vi "scan.vi"() -> ()   [LabVIEW 2017]
uses:
  tools/core/var_config.ctl
  ctrl/var_list.ctl
  tools/analysis/analysis_parameters.ctl
  tools/plotting/plot_element_2D.ctl
  tools/core/generic_config.ctl
  hardware/lecroy/scope_config.ctl
  tools/h5/data_2D.ctl
  tools/analysis/cursors.ctl
  tools/analysis/analysis_result2D.ctl
  tools/core/scan_config.ctl
  <instrlib>/LeCroy Wave Series/Public/Data/Read Multiple Waveforms.vi
  tools/tools.lvlib
  <instrlib>/LeCroy Wave Series/LeCroy Wave Series.lvlib
  hardware/lecroy/lecroy.lvlib
  hardware/highfinesse/highfinesse.lvlib
  <vilib>/gmath/NI_Gmath.lvlib
panel:
  out "state":string
  out "i_chart":dbl(graph)=808.0 caption="index chart"
  in  "preview":bool
  out "v1_chart":dbl(graph) caption="none"
  out "refresh_XY_graph":bool=TRUE
  out "v0_chart":dbl(graph)=644.7000000000019 caption="sirah_shg (nm)"
  out "scope overlay":waveform(dbl)[](graph)
  out "scope data":waveform(dbl)[](graph)
  in  "abort":bool
  in  "pause":bool
  in  "go!":bool
  in  "record":bool=TRUE
  in  "Tab Control":T1(tab)
  in  "exclude":dbl
  in  "plot_lines":bool=TRUE
  in  "sort_by_x":bool caption="sort_x"
  in  "plot_y":T2=enum."f"
  in  "plot_x":T2=enum."v0"
  out "measurement":i32(slide) caption="measurement 508 of 508" scale=0.0..508.0
  out "run_ID":string
  in  "exclude_where_x":bool caption="exclude_x"
  out "v1":dbl caption="none" format="%#_6p"
  out "v0":dbl caption="sirah_shg (nm)" format="%#_6p"
  out "XY Graph":cluster{"sorted_x":dbl[], "sorted_y ":dbl[]}[](graph)
  in  "v0_sort":bool
  in  "test0":bool caption="v0_empty"
  in  "always_update_v0":bool caption="always update?"
  in  "v0_values":dbl[](array[numeric]) format="%#_8p"
  in  "v0_config":T3={"hardware"=enum."none", "options"="", "repeats"=1, "loops"=1, "VISA"="COM9", "override_VISA"=FALSE} {"loops" min=1; "repeats" min=1}
  in  "v0_empty":bool
  in  "v0_build":bool
  in  "v0_shuffle":bool
  in  "v0_load_scan":bool
  in  "v0_save_scan":bool
  in  "v0_func":bool
  in  "v0_inject":bool
  in  "wait_after_v0 (ms)":u32 caption="wait after update (ms)"
  in  "v1_sort":bool
  in  "test1":bool caption="v0_empty"
  in  "always_update_v1":bool caption="always update?"
  in  "v1_config":T3={"hardware"=enum."none", "options"="", "repeats"=1, "loops"=1, "VISA"="COM7", "override_VISA"=FALSE} {"loops" min=1; "repeats" min=1}
  in  "v1_values":dbl[](array[numeric]) format="%#_8p"
  in  "v1_build":bool
  in  "v1_shuffle":bool
  in  "v1_load_scan":bool
  in  "v1_save_scan":bool
  in  "v1_func":bool
  in  "v1_empty":bool
  in  "v1_inject":bool
  in  "wait_after_v1 (ms)":u32 caption="wait after update (ms)"
  in  "source_w1":enum16{"None", "ch1", "ch2", "ch3", "ch4"}(ring)
  in  "source_w0":enum16{"None", "ch1", "ch2", "ch3", "ch4"}(ring)=enum."ch1"
  out "w0_chart":dbl(graph)=644.6808140624936 caption="w0"
  out "w1_chart":dbl(graph)=789.49741 caption="w0"
  in  "export_traces":bool
  in  "get_trace":bool
  out "scope display":waveform(dbl)[](graph)
  out "num_points":i32=2502 caption="points"
  out "dt":dbl=8.000000106811456e-10 format="%#_6p"
  out "num_channels":i32=2 caption="channels"
  out "position":dbl format="%#_6p"
  out "num_overlays":i32=2 caption="overlays"
  in  "wipe overlay":bool
  in  "add overlay":bool
  in  "func":string="a0 - a1" caption="f(a0, a1, a2)"
  out "f_chart":dbl(graph)=-0.0002091954192595339 caption="f (a0, a1, a2)"
  out "a2_chart":dbl(graph)=0.00039806566036490264 caption="a2"
  out "a1_chart":dbl(graph)=-0.0009949684471661708 caption="a1"
  in  "a2":T5={"source"=enum."scope 0", "window"=enum."EF", "type"=enum."mean"}
  in  "a1":T5={"source"=enum."scope 0", "window"=enum."CD", "type"=enum."mean"}
  in  "a0":T5={"source"=enum."scope 0", "window"=enum."AB", "type"=enum."mean"}
  out "a0_chart":dbl(graph)=-0.0012041638664257047 caption="a0"
  in  "scope_config":T6={"scope_VISA"="lecroy", "scope_channels"=[enum."Channel 1"], "timeout (ms)"=100000, "scope_max_points"=2500, "averages"=50} {"averages" min=1; "scope_max_points" items=["50"=50, "100"=100, "250"=250, "500"=500, "1000"=1000, "2500"=2500, "5K"=5000, "10K"=10000, "25K"=25000, "50K"=50000, "100K"=100000, "250K"=250000, "500K"=500000, "1M"=1000000, "2M"=2000000, "2.5M"=2500000, "5M"=5000000, "10M"=10000000, "25M"=25000000, "50M"=50000000, "100M"=100000000]}
  in  "scope_hold_off (ms)":u32=2000 caption="scope hold off (ms)"
  in  "auto_hold":bool=TRUE caption="super_shuffle?"
  in  "var mode":enum16{"permutations", "aligned"}(ring)
  in  "super_shuffle":bool caption="super_shuffle?"
  in  "generic settings":T7={"generic cmd"="", "upper_limit"=5.0, "lower limit"=0.05, "format"="%#.8g"} {"upper_limit" format="%#_13g"}
  in  "trigger rate (Hz)":dbl=25.0
  in  "record_vars":bool=TRUE
  in  "base":path[](array[path])=[path "C:/Users/Adam/scan_data", path "Q:/E11_atmos/scan_data"]
  out "output":path[](array[path])
  out "save_queue":i32
  in  "save_traces":bool=TRUE
  out "queue_full?":bool
  in  "exit":bool
  # "e11 scan"
  # "HighFinesse software must be running"
  # "Configure hardware using \n\n/ctrl/var_master.vi \n\nand the subVIs in \n\n/ctrl/vars"
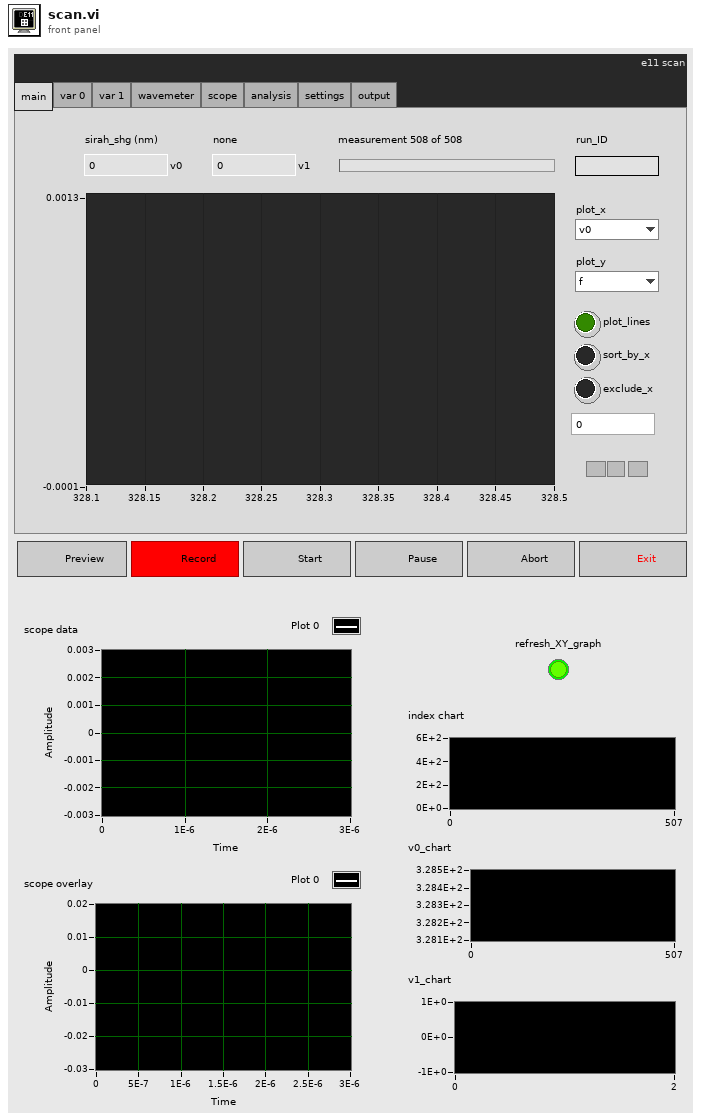
[diagram p1: front panel]
types:
  T1 = enum32{"main", "var 0", "var 1", "wavemeter", "scope", "analysis", "settings", "output"}
  T2 = typedef "tools.lvlib/plot_element_2D.ctl" = enum16{"i", "v0", "v1", "w0", "w1", "a0", "a1", "a2", "f"}
  T3 = typedef "tools.lvlib/var_config.ctl" = cluster{"hardware":T4, "options":string, "repeats":i32, "loops":i32, "VISA":refnum<visa-resource-name>, "override_VISA":bool}
  T4 = typedef "var_list.ctl" = enum16{"none", "AO voltage (V)", "delay (s)", "generic", "microwaves (GHz)", "radiant (nm)", "radiant thg (nm)", "sirah (nm)", "sirah_shg (nm)", "tenma voltage (V)", "wait (s)", "wf_freq (Hz)", "wf_amp (V)", "wf_amp_multi (V)", "wf_offset (V)", "wf_low_level (V)", "wf_high_level (V)", "wf_period (s)", "wf_pulse_width (s)", "wf_sample_rate (Sa/s)", "wf_multi_amp", "wf_multi_freq", "wf_arb_4chan", "WS7 setpoint (nm)"}
  T5 = typedef "tools.lvlib/analysis_parameters.ctl" = cluster{"source":enum16{"scope 0", "scope 1", "scope 2", "scope 3"}, "window":enum16{"AB", "CD", "EF"}, "type":enum16{"sum", "mean", "range"}}
  T6 = typedef "lecroy.lvlib/scope_config.ctl" = cluster{"scope_VISA":refnum<visa-resource-name>, "scope_channels":enum16{"Channel 1", "Channel 2", "Channel 3", "Channel 4"}[], "timeout (ms)":u32, "scope_max_points":i32, "averages":i32}
  T7 = typedef "tools.lvlib/generic_config.ctl" = cluster{"generic cmd":string, "upper_limit":dbl, "lower limit":dbl, "format":string}
  T8 = typedef "tools.lvlib/data_2D.ctl" = cluster{"files":path[], "record":bool, "save traces":bool, "raw data":waveform(dbl)[], "scope_position":dbl, "cursors":T9, "analysis_result":T10, "analysis_pars":T5[], "func":string}
  T9 = typedef "tools.lvlib/cursors.ctl" = cluster{"A":dbl, "B":dbl, "C":dbl, "D":dbl, "E":dbl, "F":dbl}
  T10 = typedef "tools.lvlib/analysis_result2D.ctl" = cluster{"v0":dbl, "v1":dbl, "w0":dbl, "w1":dbl, "a0":dbl, "a1":dbl, "a2":dbl, "f":dbl}
  T11 = enum8{"Enabled", "Disabled", "Disabled and Grayed Out"}
  T12 = enum16{"All Properties", "Averaging", "Interpolation", "Noise Filter", "Invert"}
  T13 = typedef "tools.lvlib/scan_config.ctl" = cluster{"v0 name":string, "v0 num":i32, "v1 name":string, "v1 num":i32, "scan_values":dbl[][], "num rows":i32, "measurement":i32, "v0_config":T3, "v1_config":T3}
  T14 = enum16{"Channel 1", "Channel 2", "Channel 3", "Channel 4"}[]
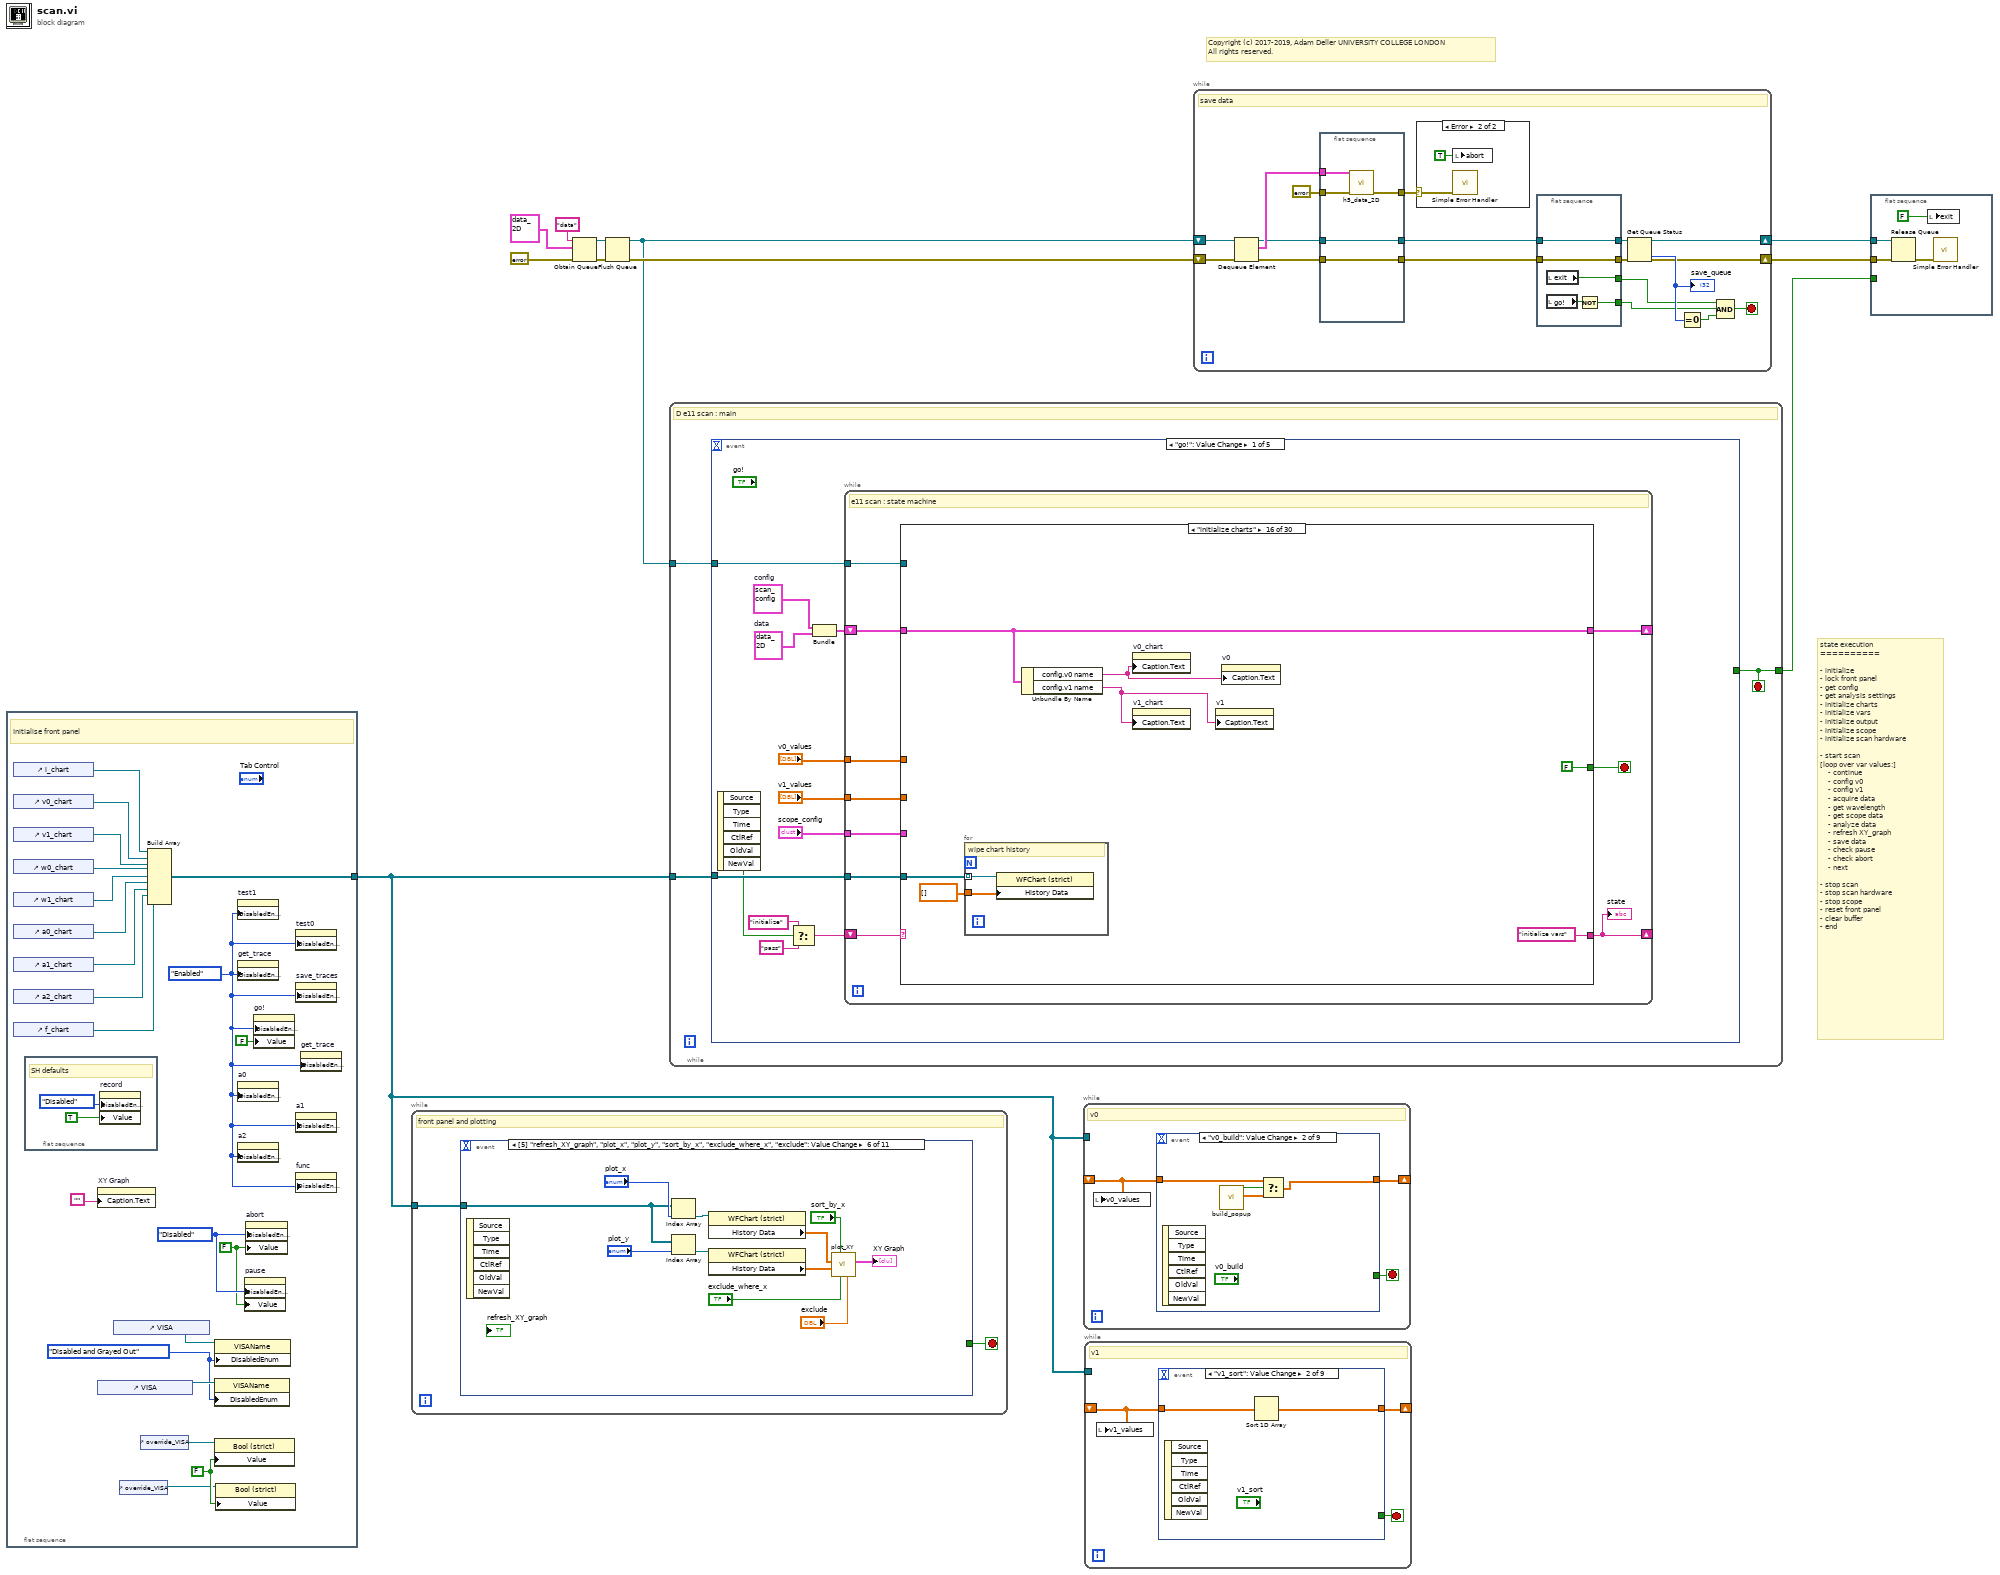
[diagram p0: block diagram]
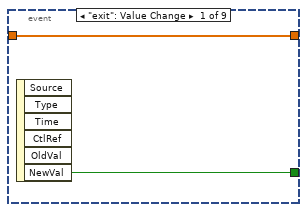
[diagram p2: hidden frame]
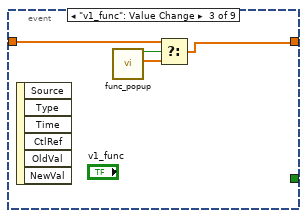
[diagram p3: hidden frame]
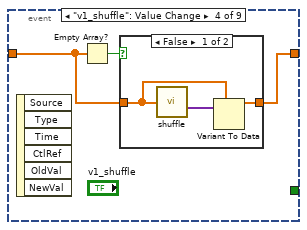
[diagram p4: hidden frame]
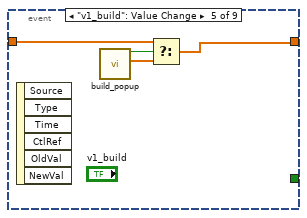
[diagram p6: hidden frame]
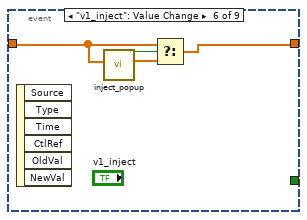
[diagram p7: hidden frame]
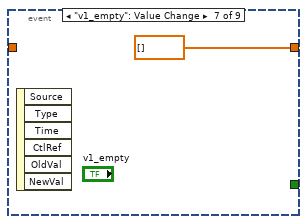
[diagram p8: hidden frame]
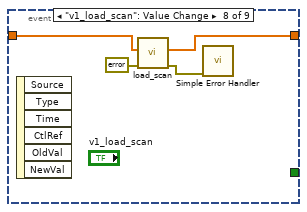
[diagram p9: hidden frame]
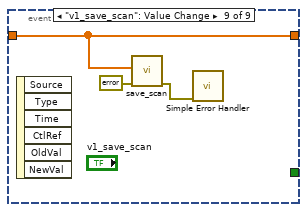
[diagram p10: hidden frame]
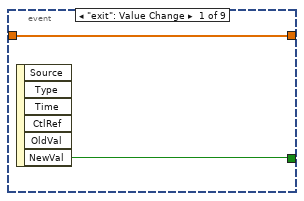
[diagram p11: hidden frame]
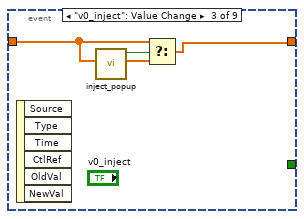
[diagram p12: hidden frame]
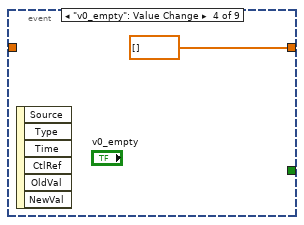
[diagram p13: hidden frame]
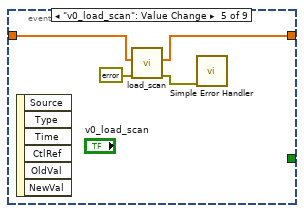
[diagram p14: hidden frame]
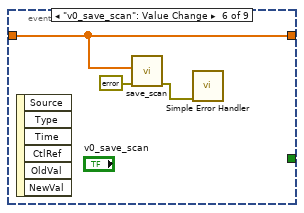
[diagram p15: hidden frame]
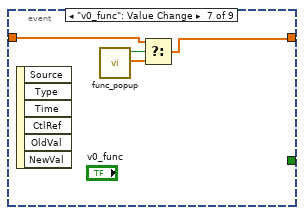
[diagram p16: hidden frame]
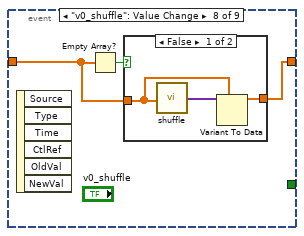
[diagram p17: hidden frame]
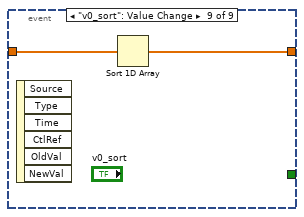
[diagram p19: hidden frame]
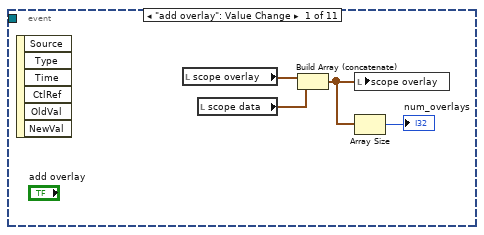
[diagram p20: hidden frame]
diagram:
  # "state execution\n==========\n\n- initialize\n- lock front panel\n- get config\n- get analysis settings\n- initialize charts\n- initialize vars\n- initialize output\n- initialize scope\n- initialize scan hardware\n\n- start scan\n[loop over var values:]\n    - continue\n    - config v0\n    - config v1\n    - acquire data\n    - get wavelength\n    - get scope data\n    - analyze data\n    - refresh XY_graph\n    - save data\n    - check pause\n    - check abort\n    - next\n\n- stop scan\n- stop scan hardware\n- stop scope\n- reset front panel\n- clear buffer\n- end"
  # "Copyright (c) 2017-2019, Adam Deller UNIVERSITY COLLEGE LONDON\nAll rights reserved."
  n1 = flat-sequence {
    tunnel: [w26] -> w1
    frame #0 {
      w17 = FALSE ("Value")
      w14 = T11."Disabled and Grayed Out" ("Disabled")
      w31 = FALSE ("abort")
      w32 = T11."Disabled" ("Disabled")
      w13 = T11."Enabled" ("Disabled")
      # "Initialise front panel"
      n2 = control-ref of="i_chart"() -> (w20:refnum<vi>)
      n3 = control-ref of="v0_chart"() -> (w22:refnum<vi>)
      n4 = control-ref of="v1_chart"() -> (w21:refnum<vi>)
      n5 = control-ref of="w0_chart"() -> (w23:refnum<vi>)
      n6 = control-ref of="w1_chart"() -> (w24:refnum<vi>)
      n7 = control-ref of="a0_chart"() -> (w27:refnum<vi>)
      n8 = control-ref of="a1_chart"() -> (w28:refnum<vi>)
      n9 = control-ref of="a2_chart"() -> (w29:refnum<vi>)
      n10 = control-ref of="f_chart"() -> (w25:refnum<vi>)
      n11 = flat-sequence {
        frame #0 {
          # "SH defaults"
          n12 = property on="record" class="Bool (strict)"("DisabledEnum"=T11."Disabled" ("Disabled"), "Value"=TRUE ("record")) -> ()  [unwired: 2 in, 2 out]
        }
      }
      n13 = property on="XY Graph" class="XYGraph (strict)"("Caption.Text"="") -> ()  [unwired: 2 in, 2 out]
      n14 = control-ref of="VISA"() -> (w15:refnum<vi>)
      n15 = control-ref of="VISA"() -> (w19:refnum<vi>)
      n16 = control-ref of="override_VISA"() -> (w16:refnum<vi>)
      n17 = control-ref of="override_VISA"() -> (w18:refnum<vi>)
      n18 = Build Array(w20, w22, w21, w23, w24, w27, w28, w29, w25) -> (w26:refnum<vi>[])
      n19 = property on="Property Node" class="VISAName"(reference=w15, "DisabledEnum"=w14) -> ()  [unwired: 1 in, 2 out]
      n20 = property on="Property Node" class="Bool (strict)"(reference=w18, "Value"=w17) -> ()  [unwired: 1 in, 2 out]
      n21 = property on="Property Node" class="VISAName"(reference=w19, "DisabledEnum"=w14) -> ()  [unwired: 1 in, 2 out]
      n22 = property on="Property Node" class="Bool (strict)"(reference=w16, "Value"=w17) -> ()  [unwired: 1 in, 2 out]
      n23 = property on="test1" class="Bool"("DisabledEnum"=w13) -> ()  [unwired: 2 in, 2 out]
      n24 = property on="get_trace" class="Bool"("DisabledEnum"=w13) -> ()  [unwired: 2 in, 2 out]
      n25 = property on="a0" class="Clust (strict)"("DisabledEnum"=w13) -> ()  [unwired: 2 in, 2 out]
      n26 = property on="a2" class="Clust (strict)"("DisabledEnum"=w13) -> ()  [unwired: 2 in, 2 out]
      n27 = property on="pause" class="Bool (strict)"("DisabledEnum"=w32, "Value"=w31) -> ()  [unwired: 2 in, 2 out]
      n28 = property on="abort" class="Bool (strict)"("DisabledEnum"=w32, "Value"=w31) -> ()  [unwired: 2 in, 2 out]
      n29 = property on="go!" class="Bool (strict)"("DisabledEnum"=w13, "Value"=FALSE ("go")) -> ()  [unwired: 2 in, 2 out]
      n30 = property on="test0" class="Bool"("DisabledEnum"=w13) -> ()  [unwired: 2 in, 2 out]
      n31 = property on="save_traces" class="Bool (strict)"("DisabledEnum"=w13) -> ()  [unwired: 2 in, 2 out]
      n32 = property on="a1" class="Clust (strict)"("DisabledEnum"=w13) -> ()  [unwired: 2 in, 2 out]
      n33 = property on="func" class="Str"("DisabledEnum"=w13) -> ()  [unwired: 2 in, 2 out]
      n34 = property on="get_trace" class="Bool"("DisabledEnum"=w13) -> ()  [unwired: 2 in, 2 out]
    }
  }
  n35 = while {
    tunnel: w1 -> [w35]
    stop <- w36 stop-if-true
    # "front panel and plotting"
    n36 = event shown="[5] \"refresh_XY_graph\", \"plot_x\", \"plot_y\", \"sort_by_x\", \"exclude_where_x\", \"exclude\": Value Change" {
      selector: _ -> [_ _ _ _ _ _ _ _ _ _ _]
      dyn-events: _ -> [_ _ _ _ _ _ _ _ _ _ _]
      timeout: _ -> [_ _ _ _ _ _ _ _ _ _ _]
      tunnel: [_ w41 _ _ _ _ _ _ _ _ _] -> w36
      tunnel: w35 -> [_ _ _ _ _ w70 _ _ _ _ _]
      event "add overlay": Value Change {
        n37 = event-data() -> ()  [unwired: 1 in, 6 out]
        n38 = local read "scope overlay"() -> (w38:waveform(dbl)[])
        n39 = local read "scope data"() -> (w37:waveform(dbl)[])
        n40 = Build Array (concatenate)(w38, w37) -> (w39:waveform(dbl)[])
        n41 = local write "scope overlay"(w39) -> ()
        n42 = Array Size(array=w39) -> (size(s)=→"num_overlays":i32)
      }
      event "exit": Value Change {
        n43 = event-data() -> ("NewVal"=w41:bool)  [unwired: 1 in, 5 out]
      }
      event "export_traces": Value Change {
        n44 = event-data() -> ()  [unwired: 1 in, 6 out]
        n45 = local read "position"() -> (w44:dbl)
        n46 = local read "scope data"() -> (w45:waveform(dbl)[])
        n47 = call "save_traces.vi"("error in"=errorcluster {"status"=FALSE, "code"=0, "source"=""}, "position"=w44, "data"=w45) -> ("error out"=w43:errorcluster)  [unwired: 8 in]
        n48 = call <vilib>:"Simple Error Handler.vi"("error in (no error)"=w43) -> ()  [unwired: 4 in, 5 out]
      }
      event "plot_lines": Value Change {
        n49 = event-data() -> ()  [unwired: 1 in, 6 out]
        n50 = case shown="True" "plot_lines" {
          tunnel: [u8 0 ("Plot.Line Style") u8 0 ("Plot.Line Style")] -> w47
          tunnel: [u8 0 u8 1 ("Plot.Line Width")] -> w48
          tunnel: [u32 16448250 ("Plot.Fill/Point Color") u32 8289918 ("Plot.Fill/Point Color")] -> w49
          tunnel: [u8 1 ("Plot.Point Style") u8 12 ("Plot.Point Style")] -> w50
          tunnel: [u32 14671839 ("Plot.Plot Color") u32 14671839 ("Plot.Plot Color")] -> w51
          tunnel: [u8 0 ("Plot.Plot Interpolation") u8 2 ("Plot.Plot Interpolation")] -> w52
          frame False {
          }
          frame True {
          }
        }
        n51 = property on="XY Graph" class="XYGraph (strict)"("Plot.Line Style"=w47, "Plot.Line Width"=w48, "Plot.Fill/Pt. Color"=w49, "Plot.Point Style"=w50, "Plot.Plot Color"=w51, "Plot.Plot Interpolation"=w52) -> ()  [unwired: 2 in, 2 out]
      }
      event "preview": Value Change {
        n52 = event-data() -> ()  [unwired: 1 in, 6 out]
        n53 = local read "v0_config"() -> (w65:T3)
        n54 = local read "v0_values"() -> (w66:dbl[])
        n55 = local read "v1_config"() -> (w67:T3)
        n56 = local read "v1_values"() -> (w68:dbl[])
        n57 = local read "var mode"() -> (w69:enum16{"permutations", "aligned"})
        n58 = call "preview_popup.vi"("var mode"=w69, "v1_values"=w68, "v1_config"=w67, "v0_values"=w66, "v0_config"=w65) -> ()  [unwired: 5 in, 2 out]
      }
      event "refresh_XY_graph", "sort_by_x", "exclude_where_x", "exclude": Value Change {
        n59 = event-data() -> ()  [unwired: 1 in, 6 out]
        n60 = Index Array(array=w70, index="plot_x") -> (element=w72:refnum<vi>)
        n61 = Index Array(array=w70, index="plot_y") -> (element=w71:refnum<vi>)
        n62 = property class="WFChart (strict)"(reference=w72) -> ("History Data"=w75:dbl[])  [unwired: 1 in, 2 out]
        n63 = property class="WFChart (strict)"(reference=w71) -> ("History Data"=w76:dbl[])  [unwired: 1 in, 2 out]
        n64 = call "plot_XY.vi"("exclude"="exclude", "exclude_where_x"="exclude_where_x", "sort_by_x"="sort_by_x", "Y_Data"=w76, "X_Data"=w75) -> ("XY Graph"=→"XY Graph":cluster{"sorted_x":dbl[], "sorted_y ":dbl[]}[])  [unwired: 6 in]
      }
      event Value Change {
        n65 = event-data() -> ()  [unwired: 1 in, 6 out]
        n66 = control-ref of="override_VISA"() -> (w82:refnum<vi>)
        n67 = property on="Property Node" class="Bool (strict)"(reference=w82, "Val(Sgnl)"=FALSE ("Value")) -> ()  [unwired: 1 in, 2 out]
      }
      event Value Change {
        n68 = event-data() -> ("NewVal"=w83:bool)  [unwired: 1 in, 5 out]
        n69 = control-ref of="VISA"() -> (w86:refnum<vi>)
        n70 = Select(t=T11."Enabled" ("Disabled"), s=w83, f=T11."Disabled and Grayed Out" ("Disabled")) -> (s? t:f=w87:T11)
        n71 = property on="Property Node" class="VISAName"(reference=w86, "DisabledEnum"=w87) -> ()  [unwired: 1 in, 2 out]
      }
      event Value Change {
        n72 = event-data() -> ()  [unwired: 1 in, 6 out]
        n73 = control-ref of="override_VISA"() -> (w89:refnum<vi>)
        n74 = property on="Property Node" class="Bool (strict)"(reference=w89, "Val(Sgnl)"=FALSE ("Value")) -> ()  [unwired: 1 in, 2 out]
      }
      event Value Change {
        n75 = event-data() -> ("NewVal"=w90:bool)  [unwired: 1 in, 5 out]
        n76 = Select(t=T11."Enabled" ("Disabled"), s=w90, f=T11."Disabled and Grayed Out" ("Disabled")) -> (s? t:f=w94:T11)
        n77 = control-ref of="VISA"() -> (w93:refnum<vi>)
        n78 = property on="Property Node" class="VISAName"(reference=w93, "DisabledEnum"=w94) -> ()  [unwired: 1 in, 2 out]
      }
      event "wipe overlay": Value Change {
        w95 = waveform(dbl)[] [] ("Waveform Data")
        n79 = event-data() -> ()  [unwired: 1 in, 6 out]
        n80 = local read "scope data"() -> (w97:waveform(dbl)[])
        n81 = local write "scope display"(w97) -> ()
        n82 = Array Size(array=w95) -> (size(s)=w96:i32)
        n83 = local write "num_overlays"(w96) -> ()
        "scope overlay" <- w95
      }
    }
  }
  n84 = Obtain Queue(name (unnamed)="data", element data type=T8 {"files"=[], "record"=FALSE, "save traces"=FALSE, "raw data"=[], "scope_position"=0.0, "cursors"={"A"=0.0, "B"=0.0, "C"=0.0, "D"=0.0, "E"=0.0, "F"=0.0}, "analysis_result"={"v0"=0.0, "v1"=0.0, "w0"=0.0, "w1"=0.0, "a0"=0.0, "a1"=0.0, "a2"=0.0, "f"=0.0}, "analysis_pars"=[], "func"="a0 - a1"} ("data"), error in (no error)=errorcluster {"status"=FALSE, "code"=0, "source"=""}) -> (queue out=w8:refnum<queue>, error out=w9:errorcluster)  [unwired: 2 in, 1 out]
  n85 = Flush Queue(queue=w8, error in (no error)=w9) -> (queue out=w5:refnum<queue>, error out=w6:errorcluster)  [unwired: 1 out]
  n86 = while {
    tunnel: w1 -> [w100]
    tunnel: w5 -> [w99]
    tunnel: [w98] -> w2
    stop <- w98 stop-if-true
    # "D e11 scan : main"
    n87 = event shown="[0] \"go!\": Value Change" {
      selector: _ -> [_ _ _ _ _]
      dyn-events: _ -> [_ _ _ _ _]
      timeout: _ -> [_ _ _ _ _]
      tunnel: [_ _ _ _ "exit"] -> w98
      tunnel: w100 -> [w112 _ _ _ _]
      tunnel: w99 -> [w111 _ _ _ w639]
      event "go!": Value Change {
        w105 = T13 {"v0 name"="radiant (nm)", "v0 num"=808, "v1 name"="none", "v1 num"=808, "scan_values"=[], "num rows"=808, "measurement"=0, "v0_config"={"hardware"=enum."radiant (nm)", "options"="", "repeats"=4, "loops"=1, "VISA"="COM9", "override_VISA"=TRUE}, "v1_config"={"hardware"=enum."radiant (nm)", "options"="", "repeats"=4, "loops"=1, "VISA"="COM9", "override_VISA"=TRUE}}  # config
        w107 = T8 {"files"=[], "record"=FALSE, "save traces"=FALSE, "raw data"=[], "scope_position"=0.0, "cursors"={"A"=0.0, "B"=0.0, "C"=0.0, "D"=0.0, "E"=0.0, "F"=0.0}, "analysis_result"={"v0"=0.0, "v1"=0.0, "w0"=0.0, "w1"=0.0, "a0"=0.0, "a1"=0.0, "a2"=0.0, "f"=0.0}, "analysis_pars"=[], "func"="a0 - a1"}  # data
        n88 = event-data() -> ("NewVal"=w110:bool)  [unwired: 1 in, 5 out]
        n89 = Select(t="initialize" ("state"), s=w110, f="pass" ("state")) -> (s? t:f=w101:string)
        n90 = Bundle("config"=w105, "data"=w107) -> (w106:cluster{"config":T13, "data":T8})  [unwired: 1 in]
        n91 = while {
          shift-right: [w115] -> _
          shift-left: w101 -> [w122]
          shift-right: [w120] -> _
          shift-left: w106 -> [w121]
          tunnel: w111 -> [w118]
          tunnel: w112 -> [w117]
          tunnel: "scope_config" -> [w116]
          tunnel: "v0_values" -> [w114]
          tunnel: "v1_values" -> [w113]
          stop <- w119 stop-if-true
          # "e11 scan : state machine"
          n92 = case shown="\"initialize charts\"" w122 {
            tunnel: ["stop scan" ("f") w129 w152 w176 "check abort" ("next") "end" ("f") w213 w248 "config v0" ("f") "" "initialize charts" ("next") "get analysis settings" ("next") w319 w337 "lock front panel" ("f") "initialize vars" ("next") w378 w416 w437 w480 "get config" ("next") w495 "" "save data" ("f") "clear buffer" ("f") "check pause" ("next") "continue" ("f") "stop scan hardware" ("f") "stop scope" ("f") "reset front panel" ("f")] -> w115
            tunnel: w121 -> [w125 w135 w156 w173 w182 w193 w210 w246 w274 w278 w297 w312 w326 w344 w354 w358 w383 w412 w424 w470 w488 w501 w510 w513 w520 w523 w535 w539 w549 w565]
            tunnel: [w125 w135 w155 w173 w182 w193 w218 w254 w274 w278 w296 w303 w325 w341 w353 w358 w373 w412 w423 w473 w488 w500 w510 w513 w520 w523 w534 w539 w549 w565] -> w120
            tunnel: [FALSE ("error?") FALSE ("error?") FALSE ("error?") FALSE ("error?") FALSE ("error?") FALSE ("error?") FALSE ("error?") FALSE ("error?") FALSE ("error?") TRUE ("error?") FALSE ("error?") FALSE ("error?") FALSE ("error?") FALSE ("error?") FALSE ("error?") FALSE ("error?") FALSE ("error?") FALSE ("error?") FALSE ("error?") FALSE ("error?") FALSE ("error?") FALSE ("error?") TRUE ("error?") FALSE ("error?") FALSE ("error?") FALSE ("error?") FALSE ("error?") FALSE ("error?") FALSE ("error?") FALSE ("error?")] -> w119
            tunnel: w118 -> [_ _ _ _ _ _ _ _ _ _ _ _ _ _ _ _ _ _ _ _ _ _ _ _ _ w527 _ _ _ _]
            tunnel: w117 -> [_ _ _ _ _ _ _ _ _ _ _ _ _ _ _ w361 _ _ _ _ _ _ _ _ _ _ _ _ _ _]
            tunnel: w116 -> [_ w128 _ _ _ _ _ _ _ _ _ _ w318 _ _ _ _ _ w429 _ _ _ _ _ _ _ _ _ _ w557]
            tunnel: w114 -> [_ _ _ _ _ _ w199 _ _ _ _ _ _ _ _ _ w370 w409 _ w459 _ _ _ _ _ _ _ _ w543 _]
            tunnel: w113 -> [_ _ _ _ _ _ _ w236 _ _ _ _ _ _ _ _ w369 w407 _ w458 _ _ _ _ _ _ _ _ w542 _]
            frame "abort", Default {
              n93 = local write "abort"(TRUE ("abort")) -> ()
            }
            frame "acquire data" {
              n94 = Unbundle By Name(w128) -> ("scope_VISA"=w127:refnum<visa-resource-name>)
              n95 = local read "scope_hold_off (ms)"() -> (w137:u32)
              n96 = call <instrlib>:"Configure Continuous Acquisition.vi"("error in (no error)"=errorcluster {"status"=FALSE, "code"=0, "source"=""}, "Continuous Acquisition Mode (T: On)"=TRUE, "VISA resource name"=w127) -> ("error out"=w139:errorcluster, "VISA resource name out"=w140:refnum<visa-resource-name>)  [unwired: 7 in]
              n97 = call "clear_sweeps.vi"("error in (no error)"=w139, "VISA resource name"=w140) -> ("error out"=w138:errorcluster)  [unwired: 8 in, 1 out]
              n98 = flat-sequence {
                tunnel: w138 -> [w142]
                tunnel: w137 -> [w143]
                tunnel: [w142] -> w136
                frame #0 {
                  n99 = Wait (ms)(milliseconds to wait=w143) -> ()  [unwired: 1 out]
                }
              }
              n100 = call <vilib>:"Simple Error Handler.vi"("error in (no error)"=w136) -> ("error?"=w130:bool)  [unwired: 4 in, 4 out]
              n101 = Select(t="abort", s=w130, f="get wavelength") -> (s? t:f=w129:string)
            }
            frame "analyze data" {
              n102 = Unbundle By Name(w156) -> ("data.func"=w153:string, "data.raw data"=w157:waveform(dbl)[], "data.analysis_pars"=w159:T5[], "data.cursors"=w149:T9)
              n103 = for {
                tunnel: w159 -> [w172] mode=indexing
                tunnel: [w171] -> w165 mode=indexing
                shift-right: [w169] -> w160
                shift-left: errorcluster {"status"=FALSE, "code"=0, "source"=""} ("error in") -> [w170]
                tunnel: w157 -> [w168]
                tunnel: w149 -> [w167]
                n104 = call "analyse.vi"("cursors"=w167, "error in"=w170, "Raw Data"=w168, "analysis_parameters"=w172) -> ("error out"=w169:errorcluster, "result"=w171:dbl)  [unwired: 6 in]
              }
              n105 = call <vilib>:"Simple Error Handler.vi"("error in (no error)"=w160) -> ("error?"=w145:bool)  [unwired: 4 in, 4 out]
              n106 = Index Array(array=w165) -> (element #1=w163:dbl, element #2=w162:dbl, element #3=w161:dbl)  [unwired: 3 in]
              "a1_chart" <- w162
              "a2_chart" <- w161
              "a0_chart" <- w163
              n107 = call <vilib>:"Eval Multi-Variable Scalar.vi"("error in (no error)"=errorcluster {"status"=FALSE, "code"=0, "source"=""}, "Variables"=string[] ["a0", "a1", "a2"], "X Values"=w165, "formula"=w153) -> ("error out"=w148:errorcluster, "y value"=w158:dbl)
              "f_chart" <- w158
              n108 = call <vilib>:"Simple Error Handler.vi"("error in (no error)"=w148) -> ("error?"=w146:bool)  [unwired: 4 in, 4 out]
              n109 = Bundle By Name(cluster=w156, "data.analysis_result.f"=w158, "data.analysis_result.a0"=w163, "data.analysis_result.a1"=w162, "data.analysis_result.a2"=w161) -> (w155:cluster{"config":T13, "data":T8})
              n110 = Or(x=w146, y=w145) -> (x .or. y?=w144:bool)
              n111 = Select(t="abort" ("next"), s=w144, f="refresh XY_graph" ("next")) -> (s? t:f=w152:string)
            }
            frame "check abort" {
              n112 = local read "exit"() -> (w180:bool)
              n113 = Compound Arithmetic op=OR("abort", w180) -> (w175:bool)
              n114 = Select(t="stop scan", s=w175, f="next" ("next")) -> (s? t:f=w176:string)
            }
            frame "check pause" {
              n115 = case shown="True" "pause" {
                frame False {
                  # "continue"
                }
                frame True {
                  # "wait to unpause or abort"
                  n116 = while {
                    stop <- w185 stop-if-true
                    n117 = local read "pause"() -> (w187:bool)
                    n118 = local read "abort"() -> (w189:bool)
                    n119 = local read "exit"() -> (w190:bool)
                    n120 = Not(x=w187) -> (.not. x?=w186:bool)
                    n121 = Wait (ms)(milliseconds to wait=u32 100) -> ()  [unwired: 1 out]
                    n122 = Compound Arithmetic op=OR(w189, w186, w190) -> (w185:bool)
                  }
                }
              }
            }
            frame "clear buffer" {
              n123 = flat-sequence {
                frame #0 {
                  n124 = Wait (ms)(milliseconds to wait=u32 100) -> ()  [unwired: 1 out]
                }
                frame #1 {
                  n125 = while {
                    stop <- w197 stop-if-true
                    n126 = local read "save_queue"() -> (w196:i32)
                    n127 = Equal To 0?(x=w196) -> (x = 0?=w197:bool)
                    n128 = Wait (ms)(milliseconds to wait=u32 100) -> ()  [unwired: 1 out]
                  }
                }
              }
            }
            frame "config v0" {
              n129 = Empty Array?(array=w199) -> (empty?=w201:bool)
              n130 = Unbundle By Name(w210) -> ("config.scan_values"=w208:dbl[][], "config.measurement"=w206:i32, "config.v0_config"=w204:T3)
              n131 = Not(x=w201) -> (.not. x?=w200:bool)
              n132 = Index Array(array=w208, index (row)=w206, index (col)=0 ("disabled index (col)")) -> (element=w205:dbl)
              n133 = Equal To 0?(x=w206) -> (x = 0?=w222:bool)
              n134 = feedback #1() -> (w211:dbl)  [unwired: 1 in]
              n135 = feedback-in #1(w205) -> ()
              n136 = Not Equal?(x=w205, y=w211) -> (x != y?=w223:bool)
              n137 = Compound Arithmetic op=OR(w223, w222, "always_update_v0") -> (w203:bool)
              n138 = And(x=w203, y=w200) -> (x .and. y?=w202:bool)
              n139 = feedback #2(0.0 ("value OUT")) -> (w219:dbl)
              n140 = case shown="True" w202 {
                tunnel: errorcluster {"status"=FALSE, "code"=0, "source"=""} ("error in (no error)") -> [w225 w231]
                tunnel: [w225 w229] -> w217
                tunnel: [w224 w230] -> w209
                tunnel: w219 -> [w224 _]
                tunnel: w205 -> [_ w227]
                tunnel: w204 -> [_ w226]
                frame False {
                  # "don't update"
                }
                frame True {
                  # "update"
                  n141 = call "var_master.vi"("generic settings"="generic settings", "error IN"=w231, "value IN"=w227, "config"=w226) -> ("error OUT"=w229:errorcluster, "value OUT"=w230:dbl)  [unwired: 6 in]
                  n142 = flat-sequence {
                    tunnel: w229 -> [_]
                    frame #0 {
                      n143 = Wait (ms)(milliseconds to wait="wait_after_v0 (ms)") -> ()  [unwired: 1 out]
                    }
                  }
                }
              }
              "v0" <- w209
              "v0_chart" <- w209
              n144 = feedback-in #2(w209) -> ()
              n145 = call <vilib>:"Simple Error Handler.vi"("error in (no error)"=w217) -> ("error?"=w214:bool)  [unwired: 4 in, 4 out]
              n146 = Bundle By Name(cluster=w210, "data.analysis_result.v0"=w209) -> (w218:cluster{"config":T13, "data":T8})
              n147 = Select(t="abort" ("next"), s=w214, f="config v1") -> (s? t:f=w213:string)
            }
            frame "config v1" {
              n148 = Empty Array?(array=w236) -> (empty?=w235:bool)
              n149 = Unbundle By Name(w246) -> ("config.scan_values"=w245:dbl[][], "config.measurement"=w242:i32, "config.v1_config"=w240:T3)
              n150 = Not(x=w235) -> (.not. x?=w234:bool)
              n151 = Index Array(array=w245, index (row)=w242, index (col)=1 ("disabled index (col)")) -> (element=w239:dbl)
              n152 = Equal To 0?(x=w242) -> (x = 0?=w257:bool)
              n153 = feedback #3() -> (w243:dbl)  [unwired: 1 in]
              n154 = feedback-in #3(w239) -> ()
              n155 = Not Equal?(x=w239, y=w243) -> (x != y?=w258:bool)
              n156 = Compound Arithmetic op=OR(w258, w257, "always_update_v1") -> (w237:bool)
              n157 = And(x=w237, y=w234) -> (x .and. y?=w238:bool)
              n158 = feedback #4(0.0 ("value OUT")) -> (w255:dbl)
              n159 = case shown="True" w238 {
                tunnel: errorcluster {"status"=FALSE, "code"=0, "source"=""} ("error in (no error)") -> [w260 w266]
                tunnel: [w260 w264] -> w253
                tunnel: [w259 w265] -> w251
                tunnel: w255 -> [w259 _]
                tunnel: w240 -> [_ w262]
                tunnel: w239 -> [_ w261]
                frame False {
                  # "don't update"
                }
                frame True {
                  # "update"
                  n160 = local read "generic settings"() -> (w263:T7)
                  n161 = call "var_master.vi"("generic settings"=w263, "error IN"=w266, "value IN"=w261, "config"=w262) -> ("error OUT"=w264:errorcluster, "value OUT"=w265:dbl)  [unwired: 6 in]
                  n162 = flat-sequence {
                    tunnel: w264 -> [_]
                    frame #0 {
                      n163 = Wait (ms)(milliseconds to wait="wait_after_v1 (ms)") -> ()  [unwired: 1 out]
                    }
                  }
                }
              }
              "v1" <- w251
              "v1_chart" <- w251
              n164 = feedback-in #4(w251) -> ()
              n165 = Bundle By Name(cluster=w246, "data.analysis_result.v1"=w251) -> (w254:cluster{"config":T13, "data":T8})
              n166 = call <vilib>:"Simple Error Handler.vi"("error in (no error)"=w253) -> ("error?"=w247:bool)  [unwired: 4 in, 4 out]
              n167 = Select(t="abort" ("next"), s=w247, f="acquire data") -> (s? t:f=w248:string)
            }
            frame "continue" {
              n168 = Unbundle By Name(w274) -> ("config.measurement"=w269:i32, "config.num rows"=w273:i32)
              n169 = To Double Precision Float(number=w269) -> (double precision float=→"i_chart":dbl)
              n170 = Increment(x=w269) -> (x+1=w268:i32)
              "measurement" <- w268
              n171 = Format Into String(format string="measurement %d of %d" ("string (\"\")"), w268, w273) -> (resulting string=w271:string)  [unwired: 2 in, 1 out]
              n172 = property on="measurement" class="Slide (strict)"("Caption.Text"=w271) -> ()  [unwired: 2 in, 2 out]
            }
            frame "end" {
            }
            frame "get analysis settings" {
              n173 = for {
                N: 6 -> [_]
                tunnel: [w299] -> w290 mode=indexing
                i -> [w300]
                # "get cursors"
                n174 = property on="scope display" class="WFGraph (strict)"("Active Cursor"=w300) -> ("Cursor.Cursor X"=w299:dbl)  [unwired: 2 in, 2 out]
              }
              n175 = Index Array(array=w290) -> (element #1=w289:dbl, element #2=w288:dbl, element #3=w287:dbl, element #4=w286:dbl, element #5=w285:dbl, element #6=w284:dbl)  [unwired: 6 in]
              n176 = Bundle(cluster=T9 {"A"=0.0, "B"=0.0, "C"=0.0, "D"=0.0, "E"=0.0, "F"=0.0} ("cursors 2"), "A"=w289, "B"=w288, "C"=w287, "D"=w286, "E"=w285, "F"=w284) -> (w281:T9)
              n177 = Build Array("a0", "a1", "a2") -> (w292:T5[])
              n178 = Bundle By Name(cluster=w297, "data.analysis_pars"=w292, "data.func"="func", "data.cursors"=w281) -> (w296:cluster{"config":T13, "data":T8})
            }
            frame "get config" {
              n179 = Bundle By Name(cluster=w312, "config.v0_config"="v0_config", "config.v1_config"="v1_config") -> (w304:cluster{"config":T13, "data":T8})
              n180 = Unbundle By Name("v0_config") -> ("hardware"=w306:T4)
              n181 = Unbundle By Name("v1_config") -> ("hardware"=w305:T4)
              n182 = property on="hardware" class="Enum (strict)"() -> ("Strings []"=w307:string[])  [unwired: 2 in, 2 out]
              n183 = Index Array(array=w307, index=w306) -> (element=w302:string)
              n184 = Index Array(array=w307, index=w305) -> (element=w301:string)
              n185 = Bundle By Name(cluster=w304, "config.v0 name"=w302, "config.v1 name"=w301) -> (w303:cluster{"config":T13, "data":T8})
            }
            frame "get scope data" {
              n186 = Unbundle By Name(w318) -> ("scope_VISA"=w317:refnum<visa-resource-name>, "scope_channels"=w316:T14, "timeout (ms)"=w315:u32)
              n187 = call-poly <instrlib>:"Read Data.vi"("error in (no error)"=errorcluster {"status"=FALSE, "code"=0, "source"=""}, "Timeout (10000 ms)"=w315, "Channels"=w316, "VISA resource name"=w317) -> ("error out"=w313:errorcluster, "Waveform Data"=w314:waveform(dbl)[])  [unwired: 5 in, 1 out]
              n188 = call <vilib>:"Simple Error Handler.vi"("error in (no error)"=w313) -> ("error?"=w320:bool)  [unwired: 4 in, 4 out]
              n189 = flat-sequence {
                tunnel: w314 -> [_]
                tunnel: [w335] -> w327
                frame #0 {
                  n190 = local read "scope overlay"() -> (w335:waveform(dbl)[])
                }
              }
              n191 = Bundle By Name(cluster=w326, "data.raw data"=w314) -> (w325:cluster{"config":T13, "data":T8})
              n192 = Array Size(array=w314) -> (size(s)=→"num_channels":i32)
              n193 = Index Array(array=w314, index=0) -> (element=w333:waveform(dbl))
              n194 = local write "scope data"(w314) -> ()
              n195 = Unbundle By Name(w333) -> ("Y"=w332:dbl[], "dt"=→"dt":dbl)
              n196 = Array Size(array=w332) -> (size(s)=→"num_points":i32)
              n197 = Build Array (concatenate)(w314, w327) -> (→"scope display":waveform(dbl)[])
              n198 = Select(t="abort" ("next"), s=w320, f="analyze data") -> (s? t:f=w319:string)
            }
            frame "get wavelength" {
              n199 = call "get_wl.vi"("error in (no error)"=errorcluster {"status"=FALSE, "code"=0, "source"=""}, "source"="source_w0") -> ("error out"=w348:errorcluster, "wl"=w343:dbl)  [unwired: 8 in]
              "w0_chart" <- w343
              n200 = call "get_wl.vi"("error in (no error)"=w348, "source"="source_w1") -> ("error out"=w347:errorcluster, "wl"=w342:dbl)  [unwired: 8 in]
              "w1_chart" <- w342
              n201 = Bundle By Name(cluster=w344, "data.analysis_result.w0"=w343, "data.analysis_result.w1"=w342) -> (w341:cluster{"config":T13, "data":T8})
              n202 = call <vilib>:"Simple Error Handler.vi"("error in (no error)"=w347) -> ("error?"=w336:bool)  [unwired: 4 in, 4 out]
              n203 = Select(t="abort" ("next"), s=w336, f="get scope data") -> (s? t:f=w337:string)
            }
            frame "initialize" {
              n204 = Bundle By Name(cluster=w354, "config.scan_values"=dbl[][] [] ("scan_values"), "config.measurement"=0 ("measurement")) -> (w353:cluster{"config":T13, "data":T8})
            }
            frame "initialize charts" {
              n205 = for {
                tunnel: w361 -> [w364] mode=indexing
                tunnel: dbl[] [] ("History Data") -> [w363]
                # "wipe chart history"
                n206 = property class="WFChart (strict)"(reference=w364, "History Data"=w363) -> ()  [unwired: 1 in, 2 out]
              }
              n207 = Unbundle By Name(w358) -> ("config.v0 name"=w356:string, "config.v1 name"=w357:string)
              n208 = property on="v0_chart" class="WFChart (strict)"("Caption.Text"=w356) -> ()  [unwired: 2 in, 2 out]
              n209 = property on="v1_chart" class="WFChart (strict)"("Caption.Text"=w357) -> ()  [unwired: 2 in, 2 out]
              n210 = property on="v1" class="DigNum (strict)"("Caption.Text"=w357) -> ()  [unwired: 2 in, 2 out]
              n211 = property on="v0" class="DigNum (strict)"("Caption.Text"=w356) -> ()  [unwired: 2 in, 2 out]
            }
            frame "initialize output" {
              n212 = Get Date/Time In Seconds() -> (seconds since 1Jan1904=w386:timestamp)
              n213 = call "build_rid_iterating.vi"("ext"="_scan.h5", "error in (no error)"=errorcluster {"status"=FALSE, "code"=0, "source"=""}, "save?"="record", "time stamp"=w386, "base"="base") -> ("error out"=w377:errorcluster, "run ID"=w375:string, "output"=w374:path[])  [unwired: 4 in]
              "run_ID" <- w375
              "output" <- w374
              n214 = call <vilib>:"Simple Error Handler.vi"("error in (no error)"=w377) -> ("error?"=w368:bool)  [unwired: 4 in, 4 out]
              n215 = Bundle By Name(cluster=w383, "data.files"=w374, "data.record"="record", "data.save traces"="save_traces") -> (w373:cluster{"config":T13, "data":T8})
              n216 = Not(x=w368) -> (.not. x?=w366:bool)
              n217 = And(x="record", y=w366) -> (x .and. y?=w365:bool)
              n218 = case shown="True" w365 {
                tunnel: w374 -> [_ w395]
                tunnel: w375 -> [_ w394]
                tunnel: w373 -> [_ w403]
                tunnel: [FALSE ("error?") w402] -> w372
                tunnel: w370 -> [_ w401]
                tunnel: w369 -> [_ w400]
                frame False {
                }
                frame True {
                  n219 = Unbundle By Name(w403) -> ("config.v0 num"=w393:i32, "config.v0_config"=w392:T3, "config.v0 name"=w391:string)
                  n220 = Unbundle By Name(w403) -> ("config.v1 name"=w390:string, "config.v1_config"=w389:T3, "config.v1 num"=w388:i32)
                  n221 = call "h5_init_2D.vi"("files"=w395, "var 0"=w391, "v0_config"=w392, "v0_num"=w393, "RID"=w394, "error in (no error)"=errorcluster {"status"=FALSE, "code"=0, "source"=""}, "var 1"=w390, "v1_config"=w389, "v1_num"=w388) -> ("error out"=w396:errorcluster)  [unwired: 6 in]
                  n222 = call "record_vars.vi"("save?"="record_vars", "error in"=w396, "var1_values"=w400, "var0_values"=w401, "output"=w395) -> ("error out"=w399:errorcluster)  [unwired: 6 in]
                  n223 = call <vilib>:"Simple Error Handler.vi"("error in (no error)"=w399) -> ("error?"=w402:bool)  [unwired: 4 in, 4 out]
                }
              }
              n224 = Or(x=w372, y=w368) -> (x .or. y?=w371:bool)
              n225 = Select(t="abort" ("next"), s=w371, f="initialize scope") -> (s? t:f=w378:string)
            }
            frame "initialize scan hardware" {
              n226 = Unbundle By Name(w412) -> ("config.v0_config"=w410:T3, "config.v1_config"=w408:T3)
              n227 = call "pre_scan.vi"("scan_values"=w409, "error in (no error)"=errorcluster {"status"=FALSE, "code"=0, "source"=""} ("error out"), "config"=w410) -> ("error out"=w404:errorcluster)  [unwired: 8 in]
              n228 = flat-sequence {
                tunnel: w408 -> [w420]
                tunnel: w407 -> [w419]
                tunnel: [w418] -> w406
                tunnel: w404 -> [_]
                frame #0 {
                  n229 = call "pre_scan.vi"("scan_values"=w419, "error in (no error)"=errorcluster {"status"=FALSE, "code"=0, "source"=""} ("error out"), "config"=w420) -> ("error out"=w418:errorcluster)  [unwired: 8 in]
                }
              }
              n230 = Merge Errors(w404, w406) -> (w405:errorcluster)
              n231 = call <vilib>:"Simple Error Handler.vi"("error in (no error)"=w405) -> ("error?"=w413:bool)  [unwired: 4 in, 4 out]
              n232 = Select(t="abort" ("next"), s=w413, f="start scan") -> (s? t:f=w416:string)
            }
            frame "initialize scope" {
              n233 = Unbundle By Name(w429) -> ("scope_max_points"=w425:i32, "scope_channels"=w426:T14, "averages"=w427:i32, "scope_VISA"=w428:refnum<visa-resource-name>)
              n234 = call <instrlib>:"Initialize.vi"("error in (no error)"=errorcluster {"status"=FALSE, "code"=0, "source"=""}, "Reset? (T: Yes)"=FALSE, "VISA resource name"=w428) -> ("error out"=w446:errorcluster, "VISA resource name out"=w445:refnum<visa-resource-name>)  [unwired: 7 in]
              n235 = call "read_position.vi"("error in (no error)"=w446, "VISA resource name"=w445) -> ("error out"=w443:errorcluster, "position (s)"=w422:dbl, "VISA resource name out"=w444:refnum<visa-resource-name>)  [unwired: 7 in]
              "position" <- w422
              n236 = call "auto_hold.vi"("averages"=w427, "trigger rate (Hz)"="trigger rate (Hz)", "hold_off"="scope_hold_off (ms)", "auto_hold"="auto_hold") -> ("hold_off (out)"=w431:u32)  [unwired: 7 in]
              n237 = Bundle By Name(cluster=w424, "data.scope_position"=w422) -> (w423:cluster{"config":T13, "data":T8})
              n238 = for {
                shift-right: [w456] -> w450
                shift-left: w443 -> [w454]
                shift-right: [w455] -> w447
                shift-left: w444 -> [w453]
                tunnel: w427 -> [w451]
                tunnel: w426 -> [w452] mode=indexing
                n239 = call <instrlib>:"Configure Channel Preprocessing.vi"("VISA resource name"=w453, "Channel (0: Channel 1)"=w452, "error in (no error)"=w454, "Sweeps to Average (1)"=w451) -> ("VISA resource name out"=w455:refnum<visa-resource-name>, "error out"=w456:errorcluster)  [unwired: 10 in]
              }
              n240 = local write "scope_hold_off (ms)"(w431) -> ()
              n241 = call "num_points.vi"("error in (no error)"=w450, "Maximum Sample Points (500)"=w425, "VISA resource name"=w447) -> ("error out"=w449:errorcluster, "VISA resource name out"=w448:refnum<visa-resource-name>)  [unwired: 7 in]
              n242 = call <instrlib>:"Configure Continuous Acquisition.vi"("error in (no error)"=w449, "Continuous Acquisition Mode (T: On)"=TRUE, "VISA resource name"=w448) -> ("error out"=w435:errorcluster)  [unwired: 7 in, 1 out]
              n243 = call <vilib>:"Simple Error Handler.vi"("error in (no error)"=w435) -> ("error?"=w434:bool)  [unwired: 4 in, 4 out]
              n244 = Select(t="abort" ("next"), s=w434, f="initialize scan hardware") -> (s? t:f=w437:string)
            }
            frame "initialize vars" {
              n245 = Unbundle By Name(w470) -> ("config.v0_config"=w468:T3, "config.v1_config"=w469:T3)
              n246 = call "scan_array_2D.vi"("v1_config"=w469, "v0_config"=w468, "error in"=errorcluster {"status"=FALSE, "code"=0, "source"=""}, "var mode"="var mode", "v1_values"=w458, "v0_values"=w459) -> ("error in (no error)"=w460:errorcluster, "scan_values"=w478:dbl[][])  [unwired: 4 in]
              n247 = call <vilib>:"Simple Error Handler.vi"("error in (no error)"=w460) -> ("error?"=w464:bool)  [unwired: 4 in, 4 out]
              n248 = Array Size(array=w458) -> (size(s)=w465:i32)
              n249 = Array Size(array=w459) -> (size(s)=w466:i32)
              n250 = case shown="True" "super_shuffle" {
                tunnel: w478 -> [w482 w484]
                tunnel: [w482 w483] -> w463
                frame False {
                }
                frame True {
                  n251 = call "shuffle_2D.vi"("Array IN"=w484) -> ("Array OUT"=w485:variant[][])
                  n252 = Variant To Data(type=w484, Variant=w485) -> (data=w483:dbl[][])  [unwired: 1 in, 1 out]
                }
              }
              n253 = Empty Array?(array=w463) -> (empty?=w462:bool)
              n254 = Array Size(array=w463) -> (size(s)=w474:i32[])
              n255 = Or(x=w462, y=w464) -> (x .or. y?=w461:bool)
              n256 = Index Array(array=w474) -> (element=w472:i32)  [unwired: 1 in]
              n257 = To Double Precision Float(number=w472) -> (double precision float=w471:dbl)
              n258 = Bundle By Name(cluster=w470, "config.scan_values"=w463, "config.num rows"=w472, "config.v0 num"=w466, "config.v1 num"=w465) -> (w473:cluster{"config":T13, "data":T8})
              n259 = property on="measurement" class="Slide (strict)"("Scale.Maximum"=w471, "Scale.Minimum"=0.0 ("Scale.Range:Minimum")) -> ()  [unwired: 2 in, 2 out]
              n260 = Select(t="abort" ("next"), s=w461, f="initialize output") -> (s? t:f=w480:string)
            }
            frame "lock front panel" {
              w489 = T11."Disabled and Grayed Out" ("Disabled")
              w490 = T11."Disabled" ("Disabled")
              w491 = T11."Enabled" ("Disabled")
              n261 = property on="pause" class="Bool (strict)"("DisabledEnum"=w491) -> ()  [unwired: 2 in, 2 out]
              n262 = property on="abort" class="Bool (strict)"("DisabledEnum"=w491) -> ()  [unwired: 2 in, 2 out]
              n263 = property on="go!" class="Bool (strict)"("DisabledEnum"=w490) -> ()  [unwired: 2 in, 2 out]
              n264 = property on="save_traces" class="Bool (strict)"("DisabledEnum"=w490) -> ()  [unwired: 2 in, 2 out]
              n265 = property on="record" class="Bool (strict)"("DisabledEnum"=w490) -> ()  [unwired: 2 in, 2 out]
              n266 = property on="a0" class="Clust (strict)"("DisabledEnum"=w489) -> ()  [unwired: 2 in, 2 out]
              n267 = property on="a2" class="Clust (strict)"("DisabledEnum"=w489) -> ()  [unwired: 2 in, 2 out]
              n268 = property on="test1" class="Bool"("DisabledEnum"=w489) -> ()  [unwired: 2 in, 2 out]
              n269 = property on="get_trace" class="Bool"("DisabledEnum"=w489) -> ()  [unwired: 2 in, 2 out]
              n270 = property on="a1" class="Clust (strict)"("DisabledEnum"=w489) -> ()  [unwired: 2 in, 2 out]
              n271 = property on="func" class="Str"("DisabledEnum"=w489) -> ()  [unwired: 2 in, 2 out]
              n272 = property on="test0" class="Bool"("DisabledEnum"=w489) -> ()  [unwired: 2 in, 2 out]
            }
            frame "next" {
              n273 = Unbundle By Name(w501) -> ("config.measurement"=w496:i32, "config.num rows"=w498:i32)
              n274 = Increment(x=w496) -> (x+1=w499:i32)
              n275 = Less?(x=w499, y=w498) -> (x < y?=w497:bool)
              n276 = case shown="True" w497 {
                tunnel: w501 -> [w503 w508]
                tunnel: [w503 w507] -> w500
                tunnel: w499 -> [_ w506]
                tunnel: [FALSE TRUE] -> w493
                frame False {
                }
                frame True {
                  n277 = Bundle By Name(cluster=w508, "config.measurement"=w506) -> (w507:cluster{"config":T13, "data":T8})
                }
              }
              n278 = Select(t="continue", s=w493, f="stop scan") -> (s? t:f=w495:string)
            }
            frame "pass" {
            }
            frame "refresh XY_graph" {
              n279 = property on="refresh_XY_graph" class="Bool (strict)"("Val(Sgnl)"=TRUE ("Value (Signaling)")) -> ()  [unwired: 2 in, 2 out]
            }
            frame "reset front panel" {
              w516 = FALSE ("go")
              w517 = T11."Disabled" ("Disabled")
              w518 = T11."Enabled" ("Disabled")
              n280 = property on="abort" class="Bool (strict)"("Value"=w516) -> ()  [unwired: 2 in, 2 out]
              n281 = property on="go!" class="Bool (strict)"("Value"=w516) -> ()  [unwired: 2 in, 2 out]
              n282 = property on="pause" class="Bool (strict)"("DisabledEnum"=w517) -> ()  [unwired: 2 in, 2 out]
              n283 = property on="abort" class="Bool (strict)"("DisabledEnum"=w517) -> ()  [unwired: 2 in, 2 out]
              n284 = property on="pause" class="Bool (strict)"("Value"=w516) -> ()  [unwired: 2 in, 2 out]
              n285 = property on="save_traces" class="Bool (strict)"("DisabledEnum"=w518) -> ()  [unwired: 2 in, 2 out]
              n286 = property on="go!" class="Bool (strict)"("DisabledEnum"=w518) -> ()  [unwired: 2 in, 2 out]
              n287 = property on="get_trace" class="Bool"("DisabledEnum"=w518) -> ()  [unwired: 2 in, 2 out]
              n288 = property on="a2" class="Clust (strict)"("DisabledEnum"=w518) -> ()  [unwired: 2 in, 2 out]
              n289 = property on="a0" class="Clust (strict)"("DisabledEnum"=w518) -> ()  [unwired: 2 in, 2 out]
              n290 = property on="test1" class="Bool"("DisabledEnum"=w518) -> ()  [unwired: 2 in, 2 out]
              n291 = property on="test0" class="Bool"("DisabledEnum"=w518) -> ()  [unwired: 2 in, 2 out]
              n292 = property on="a1" class="Clust (strict)"("DisabledEnum"=w518) -> ()  [unwired: 2 in, 2 out]
              n293 = property on="func" class="Str"("DisabledEnum"=w518) -> ()  [unwired: 2 in, 2 out]
            }
            frame "save data" {
              n294 = Unbundle By Name(w523) -> ("data"=w522:T8)
              n295 = Enqueue Element(queue=w527, element=w522, error in (no error)=errorcluster {"status"=FALSE, "code"=0, "source"=""}) -> (error out=w526:errorcluster)  [unwired: 1 in, 2 out]
              n296 = while {
                tunnel: w526 -> [_]
                stop <- w529 continue-if-true
                # "clear buffer"
                n297 = local read "save_queue"() -> (w531:i32)
                n298 = Greater?(x=w531, y=12) -> (0:w529:bool)
                "queue_full?" <- w529
                n299 = case shown="True" w529 {
                  frame False {
                  }
                  frame True {
                    n300 = Wait (ms)(milliseconds to wait=u32 100) -> ()  [unwired: 1 out]
                  }
                }
              }
              n301 = call <vilib>:"Simple Error Handler.vi"("error in (no error)"=w526) -> ()  [unwired: 4 in, 5 out]
            }
            frame "start scan" {
              n302 = Bundle By Name(cluster=w535, "config.measurement"=0 ("measurement")) -> (w534:cluster{"config":T13, "data":T8})
            }
            frame "stop scan" {
            }
            frame "stop scan hardware" {
              n303 = Unbundle By Name(w549) -> ("config.v0_config"=w547:T3, "config.v1_config"=w546:T3)
              n304 = call "post_scan.vi"("values"=w543, "error in (no error)"=errorcluster {"status"=FALSE, "code"=0, "source"=""}, "config"=w547) -> ("error out"=w541:errorcluster)  [unwired: 8 in]
              n305 = flat-sequence {
                tunnel: w546 -> [w555]
                tunnel: [w553] -> w545
                tunnel: w542 -> [w552]
                tunnel: w541 -> [_]
                frame #0 {
                  n306 = call "post_scan.vi"("values"=w552, "error in (no error)"=errorcluster {"status"=FALSE, "code"=0, "source"=""}, "config"=w555) -> ("error out"=w553:errorcluster)  [unwired: 8 in]
                }
              }
              n307 = Merge Errors(w541, w545) -> (w544:errorcluster)
              n308 = call <vilib>:"Simple Error Handler.vi"("error in (no error)"=w544) -> ()  [unwired: 4 in, 5 out]
            }
            frame "stop scope" {
              n309 = Unbundle By Name(w557) -> ("scope_VISA"=w556:refnum<visa-resource-name>)
              n310 = call <instrlib>:"Configure Continuous Acquisition.vi"("error in (no error)"=errorcluster {"status"=FALSE, "code"=0, "source"=""}, "Continuous Acquisition Mode (T: On)"=TRUE, "VISA resource name"=w556) -> ("error out"=w558:errorcluster, "VISA resource name out"=w559:refnum<visa-resource-name>)  [unwired: 7 in]
              n311 = call <instrlib>:"Close.vi"("error in (no error)"=w558, "VISA resource name"=w559) -> ("error out"=w563:errorcluster)  [unwired: 9 in]
              n312 = call <vilib>:"Simple Error Handler.vi"("error in (no error)"=w563) -> ()  [unwired: 4 in, 5 out]
            }
          }
          "state" <- w115
        }
      }
      event "get_trace": Value Change {
        n313 = event-data() -> ()  [unwired: 1 in, 6 out]
        n314 = local read "scope_config"() -> (w599:T6)
        n315 = Unbundle By Name(w599) -> ("scope_channels"=w603:T14, "timeout (ms)"=w602:u32, "scope_max_points"=w601:i32, "scope_VISA"=w600:refnum<visa-resource-name>, "averages"=w570:i32)
        n316 = property on="state" class="Str"(error in=errorcluster {"status"=FALSE, "code"=0, "source"=""} ("error in (no error)"), "Val(Sgnl)"="acquire data" ("Value (Signaling)")) -> (error out=w611:errorcluster)  [unwired: 1 in, 1 out]
        n317 = call <instrlib>:"Initialize.vi"("error in (no error)"=w611, "Reset? (T: Yes)"=FALSE, "VISA resource name"=w600) -> ("error out"=w591:errorcluster, "VISA resource name out"=w592:refnum<visa-resource-name>)  [unwired: 7 in]
        n318 = call "read_position.vi"("error in (no error)"=w591, "VISA resource name"=w592) -> ("error out"=w589:errorcluster, "position (s)"=w593:dbl, "VISA resource name out"=w590:refnum<visa-resource-name>)  [unwired: 7 in]
        n319 = call "num_points.vi"("error in (no error)"=w589, "Maximum Sample Points (500)"=w601, "VISA resource name"=w590) -> ("error out"=w605:errorcluster, "VISA resource name out"=w604:refnum<visa-resource-name>)  [unwired: 7 in]
        n320 = local read "scope_hold_off (ms)"() -> (w568:u32)
        n321 = local write "position"(w593) -> ()
        n322 = local read "trigger rate (Hz)"() -> (w569:dbl)
        n323 = for {
          tunnel: w603 -> [w615] mode=indexing
          shift-right: [w616] -> w606
          shift-left: w604 -> [w619]
          shift-right: [w617] -> w607
          shift-left: w605 -> [w618]
          tunnel: w570 -> [w614]
          n324 = call <instrlib>:"Configure Channel Preprocessing.vi"("VISA resource name"=w619, "Update (0: All Properties)"=T12."Averaging", "Channel (0: Channel 1)"=w615, "error in (no error)"=w618, "Sweeps to Average (1)"=w614) -> ("VISA resource name out"=w616:refnum<visa-resource-name>, "error out"=w617:errorcluster)  [unwired: 9 in]
        }
        n325 = local read "auto_hold"() -> (w567:bool)
        n326 = call "auto_hold.vi"("averages"=w570, "trigger rate (Hz)"=w569, "hold_off"=w568, "auto_hold"=w567) -> ("hold_off (out)"=w566:u32)  [unwired: 7 in]
        n327 = call <instrlib>:"Configure Continuous Acquisition.vi"("error in (no error)"=w607, "Continuous Acquisition Mode (T: On)"=TRUE, "VISA resource name"=w606) -> ("error out"=w585:errorcluster, "VISA resource name out"=w586:refnum<visa-resource-name>)  [unwired: 7 in]
        n328 = call "clear_sweeps.vi"("error in (no error)"=w585, "VISA resource name"=w586) -> ("error out"=w588:errorcluster, "VISA resource name out"=w587:refnum<visa-resource-name>)  [unwired: 8 in]
        n329 = local write "scope_hold_off (ms)"(w566) -> ()
        n330 = flat-sequence {
          tunnel: [w623] -> w582
          tunnel: w588 -> [w623]
          tunnel: w587 -> [w622]
          tunnel: [w622] -> w583
          tunnel: w566 -> [w621]
          frame #0 {
            n331 = Wait (ms)(milliseconds to wait=w621) -> ()  [unwired: 1 out]
          }
        }
        n332 = call-poly <instrlib>:"Read Data.vi"("error in (no error)"=w582, "Timeout (10000 ms)"=w602, "Channels"=w603, "VISA resource name"=w583) -> ("error out"=w608:errorcluster, "Waveform Data"=w609:waveform(dbl)[], "VISA resource name out"=w594:refnum<visa-resource-name>)  [unwired: 5 in]
        n333 = local read "scope overlay"() -> (w597:waveform(dbl)[])
        n334 = flat-sequence {
          tunnel: w609 -> [w613]
          tunnel: [""] -> w610
          frame #0 {
            "scope data" <- w613
          }
        }
        n335 = call <instrlib>:"Configure Continuous Acquisition.vi"("error in (no error)"=w608, "Continuous Acquisition Mode (T: On)"=TRUE, "VISA resource name"=w594) -> ("error out"=w596:errorcluster, "VISA resource name out"=w595:refnum<visa-resource-name>)  [unwired: 7 in]
        n336 = Index Array(array=w609, index=0) -> (element=w578:waveform(dbl))
        n337 = Array Size(array=w609) -> (size(s)=w577:i32)
        n338 = Unbundle By Name(w578) -> ("Y"=w579:dbl[], "dt"=w581:dbl)
        n339 = local write "num_channels"(w577) -> ()
        n340 = call <instrlib>:"Close.vi"("error in (no error)"=w596, "VISA resource name"=w595) -> ("error out"=w584:errorcluster)  [unwired: 9 in]
        n341 = property on="state" class="Str"("Val(Sgnl)"=w610) -> ()  [unwired: 2 in, 2 out]
        n342 = Build Array (concatenate)(w609, w597) -> (w598:waveform(dbl)[])
        n343 = local write "dt"(w581) -> ()
        n344 = Array Size(array=w579) -> (size(s)=w580:i32)
        n345 = call <vilib>:"Simple Error Handler.vi"("error in (no error)"=w584) -> ()  [unwired: 4 in, 5 out]
        n346 = local write "scope display"(w598) -> ()
        n347 = local write "num_points"(w580) -> ()
      }
      event "test0": Value Change {
        n348 = event-data() -> ()  [unwired: 1 in, 6 out]
        n349 = property on="v0_values" class="Arr (strict)"() -> ("Value"=w629:dbl[], "Index Values"=w628:u32[])  [unwired: 2 in, 2 out]
        n350 = local read "generic settings"() -> (w625:T7)
        n351 = local read "v0_config"() -> (w624:T3)
        n352 = Index Array(array=w628) -> (element=w627:u32)  [unwired: 1 in]
        n353 = Index Array(array=w629, index=w627) -> (element=w626:dbl)
        n354 = call "test_popup.vi"("value"=w626, "config"=w624, "generic settings"=w625) -> ()  [unwired: 8 in, 1 out]
      }
      event "test1": Value Change {
        n355 = event-data() -> ()  [unwired: 1 in, 6 out]
        n356 = property on="v1_values" class="Arr (strict)"() -> ("Value"=w635:dbl[], "Index Values"=w634:u32[])  [unwired: 2 in, 2 out]
        n357 = local read "generic settings"() -> (w631:T7)
        n358 = local read "v1_config"() -> (w630:T3)
        n359 = Index Array(array=w634) -> (element=w633:u32)  [unwired: 1 in]
        n360 = Index Array(array=w635, index=w633) -> (element=w632:dbl)
        n361 = call "test_popup.vi"("value"=w632, "config"=w630, "generic settings"=w631) -> ()  [unwired: 8 in, 1 out]
      }
      event "exit": Value Change {
        n362 = event-data() -> ()  [unwired: 1 in, 6 out]
        n363 = Enqueue Element(queue=w639, element=T8 {"files"=[], "record"=FALSE, "save traces"=FALSE, "raw data"=[], "scope_position"=0.0, "cursors"={"A"=0.0, "B"=0.0, "C"=0.0, "D"=0.0, "E"=0.0, "F"=0.0}, "analysis_result"={"v0"=0.0, "v1"=0.0, "w0"=0.0, "w1"=0.0, "a0"=0.0, "a1"=0.0, "a2"=0.0, "f"=0.0}, "analysis_pars"=[], "func"="a0 - a1"}, error in (no error)=errorcluster {"status"=FALSE, "code"=0, "source"=""}) -> (error out=w637:errorcluster)  [unwired: 1 in, 2 out]
        n364 = call <vilib>:"Simple Error Handler.vi"("error in (no error)"=w637) -> ()  [unwired: 4 in, 5 out]
      }
    }
  }
  n365 = while {
    shift-right: [w642] -> _
    shift-left: _ -> [w641]
    tunnel: w1 -> [_]
    stop <- w643 stop-if-true
    # "v0"
    n366 = local write "v0_values"(w641) -> ()
    n367 = event shown="[1] \"v0_build\": Value Change" {
      selector: _ -> [_ _ _ _ _ _ _ _ _]
      dyn-events: _ -> [_ _ _ _ _ _ _ _ _]
      timeout: _ -> [_ _ _ _ _ _ _ _ _]
      tunnel: [w645 _ _ _ _ _ _ _ _] -> w643
      tunnel: [w644 w646 w650 dbl[] [] ("v0_values") w657 w659 w662 w666 w673] -> w642
      tunnel: w641 -> [w644 w647 w651 _ w658 w659 w665 w667 w674]
      event "exit": Value Change {
        n368 = event-data() -> ("NewVal"=w645:bool)  [unwired: 1 in, 5 out]
      }
      event "v0_build": Value Change {
        n369 = event-data() -> ()  [unwired: 1 in, 6 out]
        n370 = call "build_popup.vi"() -> ("y_vals"=w648:dbl[], "cancelled"=w649:bool)  [unwired: 10 in]
        n371 = Select(t=w647, s=w649, f=w648) -> (s? t:f=w646:dbl[])
      }
      event "v0_inject": Value Change {
        n372 = event-data() -> ()  [unwired: 1 in, 6 out]
        n373 = call "inject_popup.vi"("y_vals_IN"=w651) -> ("y_vals"=w653:dbl[], "cancelled"=w652:bool)  [unwired: 9 in]
        n374 = Select(t=w651, s=w652, f=w653) -> (s? t:f=w650:dbl[])
      }
      event "v0_empty": Value Change {
        n375 = event-data() -> ()  [unwired: 1 in, 6 out]
      }
      event "v0_load_scan": Value Change {
        n376 = event-data() -> ()  [unwired: 1 in, 6 out]
        n377 = call "load_scan.vi"("error in"=errorcluster {"status"=FALSE, "code"=0, "source"=""}, "values in"=w658) -> ("error out"=w656:errorcluster, "values out"=w657:dbl[])  [unwired: 8 in]
        n378 = call <vilib>:"Simple Error Handler.vi"("error in (no error)"=w656) -> ()  [unwired: 4 in, 5 out]
      }
      event "v0_save_scan": Value Change {
        n379 = event-data() -> ()  [unwired: 1 in, 6 out]
        n380 = call "save_scan.vi"("error in"=errorcluster {"status"=FALSE, "code"=0, "source"=""}, "values in"=w659) -> ("error out"=w660:errorcluster)  [unwired: 9 in]
        n381 = call <vilib>:"Simple Error Handler.vi"("error in (no error)"=w660) -> ()  [unwired: 4 in, 5 out]
      }
      event "v0_func": Value Change {
        n382 = event-data() -> ()  [unwired: 1 in, 6 out]
        n383 = call "func_popup.vi"() -> ("y_vals"=w663:dbl[], "cancelled"=w664:bool)  [unwired: 10 in]
        n384 = Select(t=w665, s=w664, f=w663) -> (s? t:f=w662:dbl[])
      }
      event "v0_shuffle": Value Change {
        n385 = event-data() -> ()  [unwired: 1 in, 6 out]
        n386 = Empty Array?(array=w667) -> (empty?=w668:bool)
        n387 = case shown="False" w668 {
          tunnel: w667 -> [w670 w672]
          tunnel: [w669 w672] -> w666
          frame False {
            n388 = call "shuffle.vi"("Array IN"=w670) -> ("Array OUT"=w671:variant[])
            n389 = Variant To Data(type=w670, Variant=w671) -> (data=w669:dbl[])  [unwired: 1 in, 1 out]
          }
          frame True {
          }
        }
      }
      event "v0_sort": Value Change {
        n390 = event-data() -> ()  [unwired: 1 in, 6 out]
        n391 = Sort 1D Array(array=w674) -> (sorted array=w673:dbl[])
      }
    }
  }
  n392 = while {
    shift-right: [w675] -> _
    shift-left: _ -> [w676]
    tunnel: w1 -> [_]
    stop <- w677 stop-if-true
    # "v1"
    n393 = local write "v1_values"(w676) -> ()
    n394 = event shown="[1] \"v1_sort\": Value Change" {
      selector: _ -> [_ _ _ _ _ _ _ _ _]
      dyn-events: _ -> [_ _ _ _ _ _ _ _ _]
      timeout: _ -> [_ _ _ _ _ _ _ _ _]
      tunnel: [w679 _ _ _ _ _ _ _ _] -> w677
      tunnel: w676 -> [w678 w681 w685 w687 w694 w698 _ w703 w706]
      tunnel: [w678 w680 w682 w686 w693 w697 dbl[] [] ("v1_values") w702 w706] -> w675
      event "exit": Value Change {
        n395 = event-data() -> ("NewVal"=w679:bool)  [unwired: 1 in, 5 out]
      }
      event "v1_sort": Value Change {
        n396 = event-data() -> ()  [unwired: 1 in, 6 out]
        n397 = Sort 1D Array(array=w681) -> (sorted array=w680:dbl[])
      }
      event "v1_func": Value Change {
        n398 = event-data() -> ()  [unwired: 1 in, 6 out]
        n399 = call "func_popup.vi"() -> ("y_vals"=w684:dbl[], "cancelled"=w683:bool)  [unwired: 10 in]
        n400 = Select(t=w685, s=w683, f=w684) -> (s? t:f=w682:dbl[])
      }
      event "v1_shuffle": Value Change {
        n401 = event-data() -> ()  [unwired: 1 in, 6 out]
        n402 = Empty Array?(array=w687) -> (empty?=w688:bool)
        n403 = case shown="False" w688 {
          tunnel: w687 -> [w690 w692]
          tunnel: [w689 w692] -> w686
          frame False {
            n404 = call "shuffle.vi"("Array IN"=w690) -> ("Array OUT"=w691:variant[])
            n405 = Variant To Data(type=w690, Variant=w691) -> (data=w689:dbl[])  [unwired: 1 in, 1 out]
          }
          frame True {
          }
        }
      }
      event "v1_build": Value Change {
        n406 = event-data() -> ()  [unwired: 1 in, 6 out]
        n407 = call "build_popup.vi"() -> ("y_vals"=w696:dbl[], "cancelled"=w695:bool)  [unwired: 10 in]
        n408 = Select(t=w694, s=w695, f=w696) -> (s? t:f=w693:dbl[])
      }
      event "v1_inject": Value Change {
        n409 = event-data() -> ()  [unwired: 1 in, 6 out]
        n410 = call "inject_popup.vi"("y_vals_IN"=w698) -> ("y_vals"=w700:dbl[], "cancelled"=w699:bool)  [unwired: 9 in]
        n411 = Select(t=w698, s=w699, f=w700) -> (s? t:f=w697:dbl[])
      }
      event "v1_empty": Value Change {
        n412 = event-data() -> ()  [unwired: 1 in, 6 out]
      }
      event "v1_load_scan": Value Change {
        n413 = event-data() -> ()  [unwired: 1 in, 6 out]
        n414 = call "load_scan.vi"("error in"=errorcluster {"status"=FALSE, "code"=0, "source"=""}, "values in"=w703) -> ("error out"=w705:errorcluster, "values out"=w702:dbl[])  [unwired: 8 in]
        n415 = call <vilib>:"Simple Error Handler.vi"("error in (no error)"=w705) -> ()  [unwired: 4 in, 5 out]
      }
      event "v1_save_scan": Value Change {
        n416 = event-data() -> ()  [unwired: 1 in, 6 out]
        n417 = call "save_scan.vi"("error in"=errorcluster {"status"=FALSE, "code"=0, "source"=""}, "values in"=w706) -> ("error out"=w707:errorcluster)  [unwired: 9 in]
        n418 = call <vilib>:"Simple Error Handler.vi"("error in (no error)"=w707) -> ()  [unwired: 4 in, 5 out]
      }
    }
  }
  n419 = while {
    shift-right: [w721] -> w3
    shift-left: w5 -> [w724]
    shift-right: [w720] -> w4
    shift-left: w6 -> [w725]
    stop <- w719 stop-if-true
    # "save data"
    n420 = Dequeue Element(queue=w724, error in (no error)=w725) -> (queue out=w714:refnum<queue>, element=w715:T8, error out=w711:errorcluster)  [unwired: 1 in, 1 out]
    n421 = flat-sequence {
      tunnel: w715 -> [w730]
      tunnel: w714 -> [w733]
      tunnel: [w733] -> w713
      tunnel: [w732] -> w712
      tunnel: w711 -> [w732]
      tunnel: errorcluster {"status"=FALSE, "code"=0, "source"=""} ("error in (no error)") -> [w731]
      tunnel: [w729] -> w709
      frame #0 {
        n422 = call "h5_data_2D.vi"("error in (no error)"=w731, "data"=w730) -> ("error out"=w729:errorcluster)  [unwired: 9 in]
      }
    }
    n423 = case shown="Error" w709 {
      selector: w709 -> [_ w728]
      frame No Error {
      }
      frame Error {
        n424 = local write "abort"(TRUE ("abort")) -> ()
        n425 = call <vilib>:"Simple Error Handler.vi"("error in (no error)"=w728) -> ()  [unwired: 4 in, 5 out]
      }
    }
    n426 = flat-sequence {
      tunnel: w713 -> [w737]
      tunnel: [w738] -> w716
      tunnel: [w737] -> w722
      tunnel: [w734] -> w723
      tunnel: [w735] -> w717
      tunnel: w712 -> [w734]
      frame #0 {
        n427 = local read "exit"() -> (w738:bool)
        n428 = local read "go!"() -> (w736:bool)
        n429 = Not(x=w736) -> (.not. x?=w735:bool)
      }
    }
    n430 = Get Queue Status(queue=w722, error in (no error)=w723) -> (queue out=w721:refnum<queue>, error out=w720:errorcluster, # elements in queue=w726:i32)  [unwired: 1 in, 5 out]
    "save_queue" <- w726
    n431 = Equal To 0?(x=w726) -> (x = 0?=w718:bool)
    n432 = Compound Arithmetic op=AND(w716, w717, w718) -> (w719:bool)
  }
  n433 = flat-sequence {
    tunnel: w4 -> [w741]
    tunnel: w3 -> [w740]
    tunnel: w2 -> [_]
    frame #0 {
      n434 = Release Queue(queue=w740, error in (no error)=w741) -> (error out=w742:errorcluster)  [unwired: 1 in, 2 out]
      n435 = local write "exit"(FALSE ("exit")) -> ()
      n436 = call <vilib>:"Simple Error Handler.vi"("error in (no error)"=w742) -> ()  [unwired: 4 in, 5 out]
    }
  }
